vi "Next Step.vi"(8 "error in (no error)":errorcluster, 11 "Wavelength.lvclass in":refnum<class "Wavelength.lvclass">) -> (0 "error out":errorcluster, 1 "Step #":u32, 2 "Actual position":dbl, 3 "Wavelength.lvclass out":refnum<class "Wavelength.lvclass">)   [LabVIEW 2009, in "Wavelength.lvclass"]
uses:
  Wavelength.lvclass
  Scanner/Scanner.lvclass
  Instruments/Utility Classes/Scannable/Scannable.lvclass
  Instruments/Spectrometer/JY-SPEX-TRIAX/JY-SPEX-TRIAX.lvlib
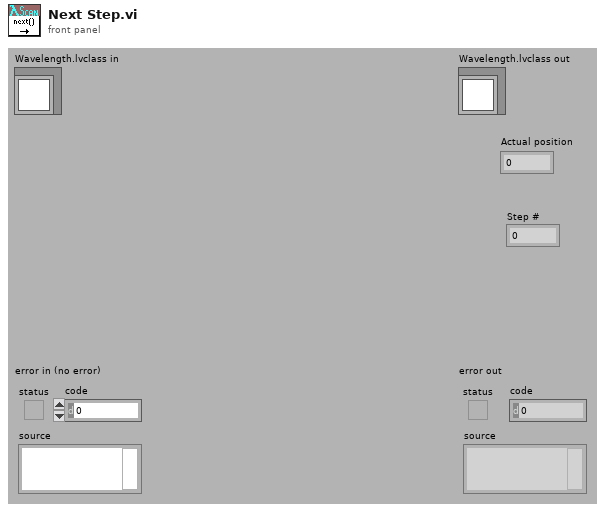
[diagram p1: front panel]
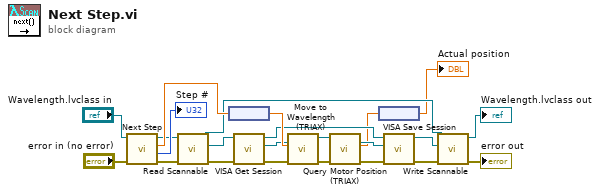
[diagram p0: block diagram]
diagram:
  n1 = call-parent "Next Step.vi"("error in (no error)"="error in (no error)", "Scanner in"="Wavelength.lvclass in") -> ("error out"=w18:errorcluster, "Current Step"=→"Step #":u32, "Current Position"=w17:dbl, "Scanner out"=w7:refnum<class "Wavelength.lvclass">)  [unwired: 1 in, 5 out]
  n2 = call-dynamic "Read Scannable.vi"("error in (no error)"=w18, "Scanner.lvclass in"=w7) -> ("error out"=w20:errorcluster, "Scannable.lvclass"=w9:refnum<class "Scannable.lvclass">, "Scanner.lvclass out"=w8:refnum<class "Wavelength.lvclass">)  [unwired: 7 out]
  n3 = node(w17) -> (w16:dbl[unit])
  n4 = call-dynamic "VISA Get Session.vi"("error in (no error)"=w20, "Instrument.lvclass in"=w9) -> ("error out"=w13:errorcluster, "VISA Resource Name"=w15:refnum<visa-resource-name>, "Instrument.lvclass out"=w14:refnum<class "Scannable.lvclass">)  [unwired: 7 out]
  n5 = call "Move to Wavelength (TRIAX).vi"("error in (no error)"=w13, "Target wavelength"=w16, "VISA resource name"=w15) -> ("error out"=w4:errorcluster, "VISA resource name out"=w12:refnum<visa-resource-name>)  [unwired: 1 in, 6 out]
  n6 = call "Query Motor Position (TRIAX).vi"("error in (no error)"=w4, "VISA resource name"=w12) -> ("error out"=w3:errorcluster, "wavelength"=w5:dbl[unit], "VISA resource name out"=w11:refnum<visa-resource-name>)  [unwired: 1 in, 6 out]
  n7 = node(w5) -> (→"Actual position":dbl)
  n8 = call-dynamic "VISA Save Session.vi"("error in (no error)"=w3, "VISA Resource Name"=w11, "Instrument.lvclass in"=w14) -> ("error out"=w19:errorcluster, "Instrument.lvclass out"=w10:refnum<class "Scannable.lvclass">)  [unwired: 7 out]
  n9 = call-dynamic "Write Scannable.vi"("error in (no error)"=w19, "Scannable.lvclass"=w10, "Scanner.lvclass in"=w8) -> ("error out"=→"error out":errorcluster, "Scanner.lvclass out"=→"Wavelength.lvclass out":refnum<class "Wavelength.lvclass">)  [unwired: 7 out]
